vi "Shut Down Device.vi"(8 "error in (no error)":errorcluster, 11 "Cobolt in":refnum<class "Cobolt Laser.lvclass">) -> (0 "error out":errorcluster, 3 "Cobolt out":refnum<class "Cobolt Laser.lvclass">)   [LabVIEW 2023, in "Cobolt Laser.lvlib" / "Cobolt Laser.lvclass"]
uses:
  Cobolt Laser.lvclass
  Laser/Laser.lvclass
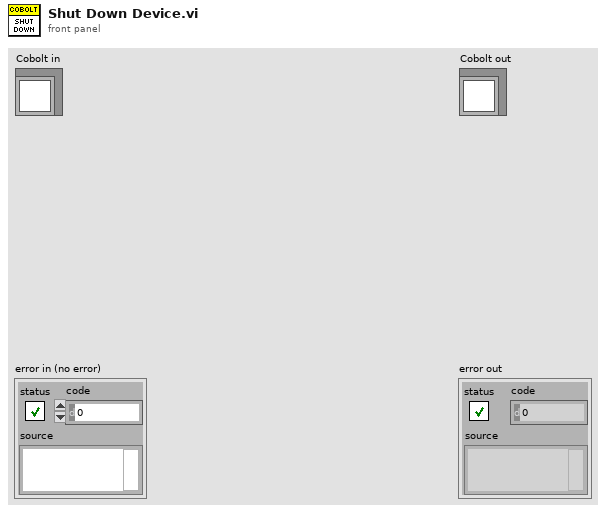
[diagram p1: front panel]
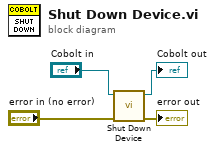
[diagram p0: block diagram]
diagram:
  n1 = call-parent "Shut Down Device.vi"("error in (no error)"="error in (no error)", "Device in"="Cobolt in") -> ("error out"=→"error out":errorcluster, "Device out"=→"Cobolt out":refnum<class "Cobolt Laser.lvclass">)  [unwired: 8 in]
